vi "Pace_value_search_high_side.vi"(9 "y":dbl, 11 "data":dbl[](array[numeric])) -> (3 "x":i32)   [LabVIEW 2016]
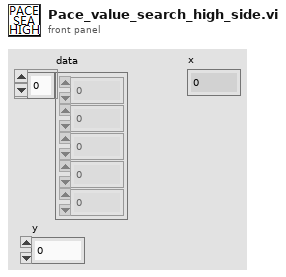
[diagram p1: front panel]
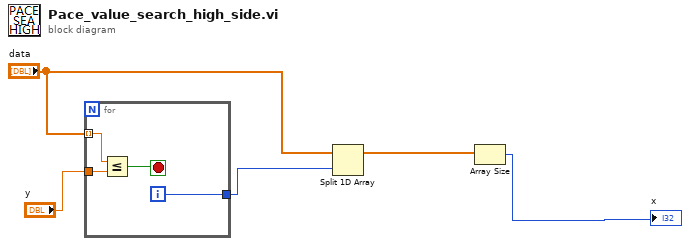
[diagram p0: block diagram]
diagram:
  n1 = for {
    tunnel: "data" -> [w9] mode=indexing
    tunnel: "y" -> [w8]
    tunnel: [w6] -> w3
    i -> [w6]
    stop <- w7 stop-if-true
    n2 = Less Or Equal?(x=w9, y=w8) -> (x <= y?=w7:bool)
  }
  n3 = Split 1D Array(array="data", index=w3) -> (first subarray=w1:dbl[])  [unwired: 1 out]
  n4 = Array Size(array=w1) -> (size(s)=→"x":i32)
